vi "NI_9222_Anologue_DAQ2_FPGA_Host.vi"() -> ()   [LabVIEW 2013]
uses:
  <vilib>/rvi/interface/nirviOpenFPGA/nirviOpenFPGA.xnode
  <vilib>/rvi/interface/nirviReadWriteControl/nirviReadWriteControl.xnode
  <vilib>/rvi/interface/Simulation/niFpgaSimulationCallBeginRW.vi
  <vilib>/rvi/errors/niLvFpgaAdjustHostInterfaceError.vi
  <vilib>/rvi/interface/nirviMethod/nirviMethod.xnode
  <vilib>/rvi/errors/niLvFpgaMergeErrorWithErrorCode.vi
  <vilib>/rvi/interface/nirviCloseFPGA/nirviCloseFPGA.xnode
  <vilib>/FPGAPlugInAG/Dynamic/niLvFpga_AcknowledgeIrq_Dynamic.vi
  <vilib>/Utility/error.llb/Error Cluster From Error Code.vi
  NiFpgaLv.dll
  <vilib>/FPGAPlugInAG/Dynamic/niLvFpga_ReadFifo_Dynamic.vi
  <vilib>/rvi/interface/nirviMethod/StockFPGA_InlinedMethodWaitForSingleIRQ.vi
  <vilib>/FPGAPlugInAG/Dynamic/niLvFpga_WaitOnIrq_Dynamic.vi
  <vilib>/FPGAPlugInAG/Dynamic/niLvFpga_StartFifo_Dynamic.vi
  <vilib>/FPGAPlugInAG/Dynamic/niLvFpga_Close_Dynamic.vi
  FPGA Bitfiles/cRioProject1_FPGATarget_NI9222AnologueDA_SSoRp+cfeGo.lvbitx
  NI_9222_Anologue_DAQ2_FPGA.vi
  <vilib>/FPGAPlugInAG/cRIO-9068/niLvFpga_Open_cRIO-9068.vi
  <vilib>/rvi/interface/common/dynamic/niFpgaDynamicAddResources.vi
  <vilib>/userdefined/High Color/nirio_resource_hc.ctl
panel:
  out "Array":i16[][](array[numeric])
  out "Array Out of FIFO size":i32[](array[numeric])
  out "Array to write size":i32[](array[numeric])
  out "Number of while loop iterations":i32
  out "time string":string
  out "Elements Remaining":u32
  out "FPGA Error Out 2":errorcluster
  out "FPGA Stop":bool
  in  "RIO Device":T1="RIO0"
  out "Timed Out":bool
  out "Sample Gated":bool
  out "Overwrite":bool
  in  "stop":bool
  in  "Sample Period (uSec)":u32=2
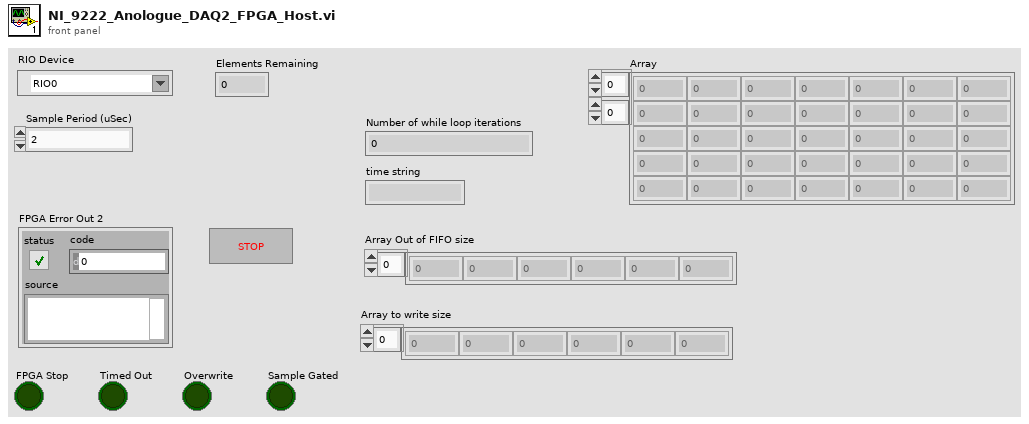
[diagram p1: front panel]
types:
  T1 = typedef "nirio_resource_hc.ctl" = tag
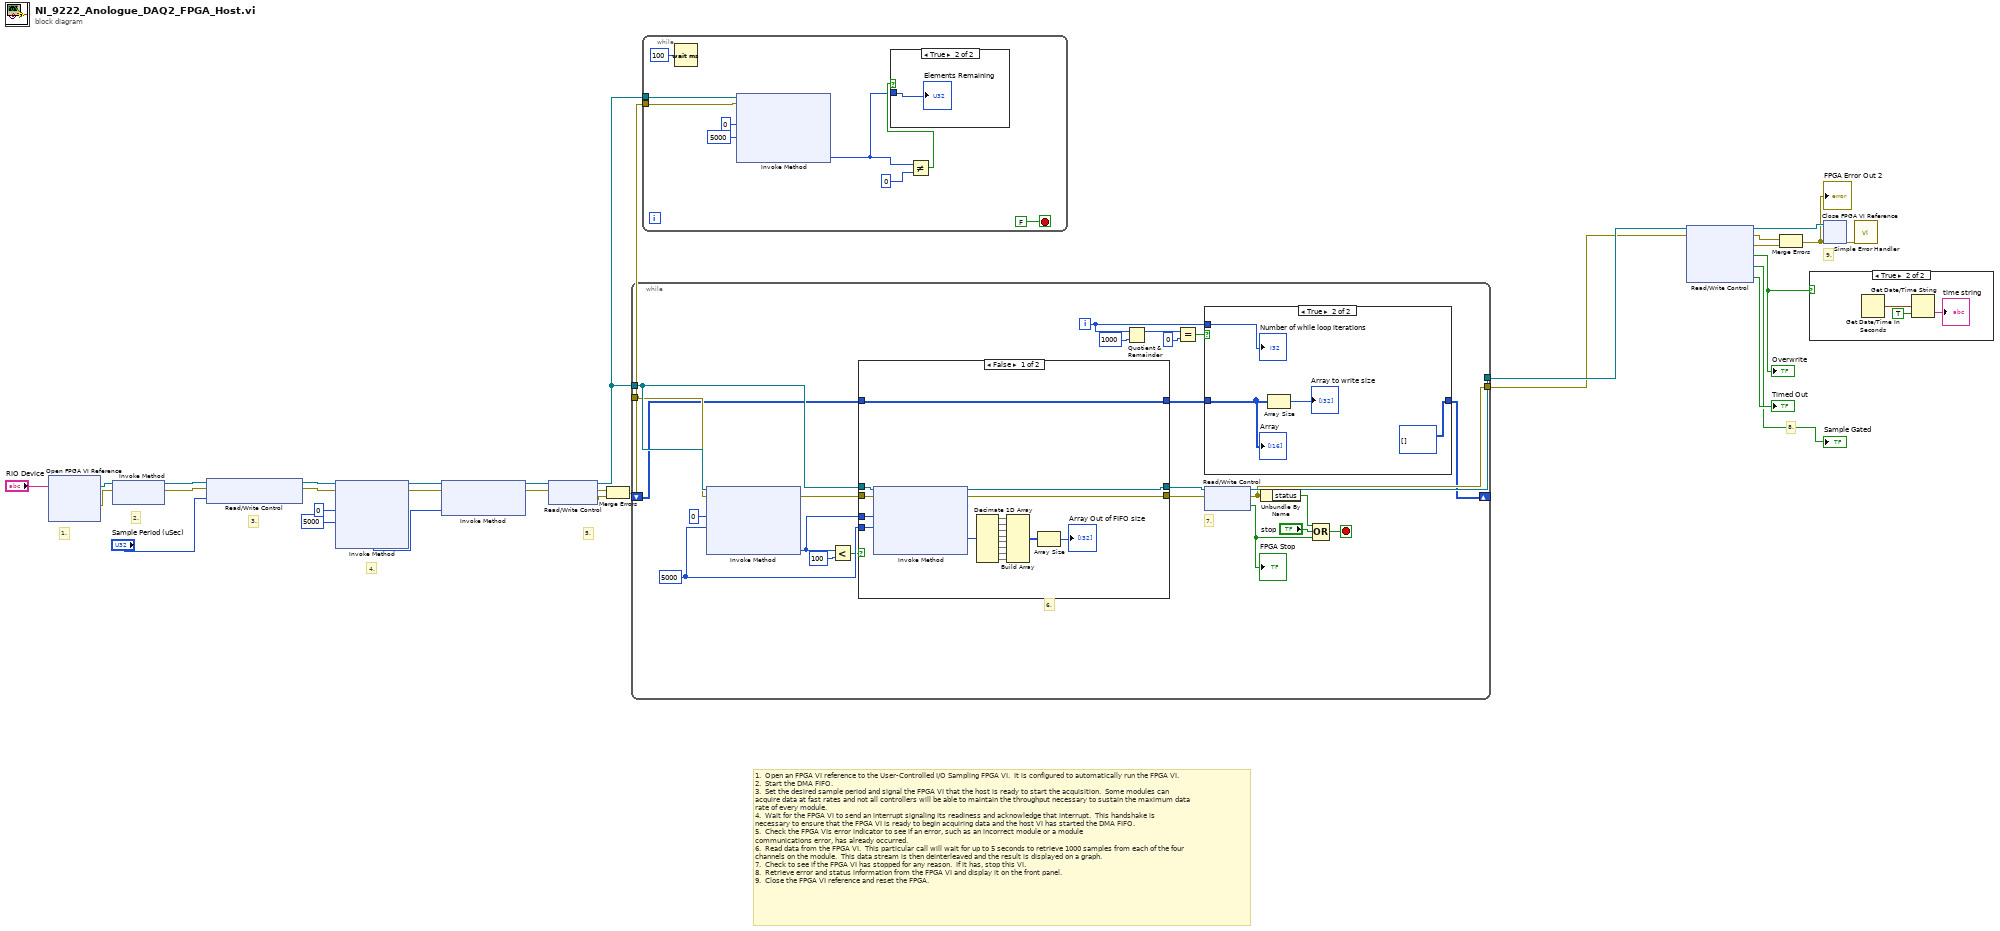
[diagram p0: block diagram]
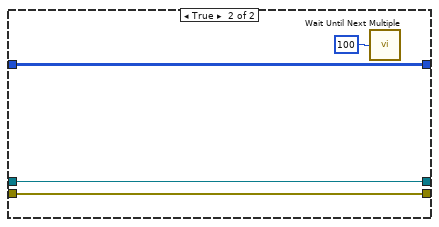
[diagram p5: hidden frame]
diagram:
  # "5."
  # "4."
  # "1.  Open an FPGA VI reference to the User-Controlled I/O Sampling FPGA VI.  It is configured to automatically run the FPGA VI.\n2.  Start the DMA FIFO.\n3.  Set the desired sample period and signal the FPGA VI that the host is ready to start the acquisition.  Some modules can \nacquire data at fast rates and not all controllers will be able to maintain the throughput necessary to sustain the maximum data \nrate of every module.\n4.  Wait for the FPGA VI to send an interrupt signaling its readiness and acknowledge that interrupt.  This handshake is \nnecessary to ensure that the FPGA VI is ready to begin acquiring data and the host VI has started the DMA FIFO.\n5.  Check the FPGA VIs error indicator to see if an error, such as an incorrect module or a module \ncommunications error, has already occurred.\n6.  Read data from the FPGA VI.  This particular call will wait for up to 5 seconds to retrieve 1000 samples from each of the four \nchannels on the module.  This data stream is then deinterleaved and the result is displayed on a graph.\n7.  Check to see if the FPGA VI has stopped for any reason.  If it has, stop this VI.\n8.  Retrieve error and status information from the FPGA VI and display it on the front panel.\n9.  Close the FPGA VI reference and reset the FPGA."
  # "9."
  # "8."
  # "3."
  # "2."
  # "1."
  n1 = xnode "Open FPGA VI Reference"("resource name"="RIO Device") -> ("FPGA VI Reference Out"=w27:refnum<k20>, "error out"=w28:errorcluster)  [unwired: 1 in]
  n2 = xnode "Invoke Method"("FPGA VI Reference In"=w27, "error in"=w28) -> ("FPGA VI Reference Out"=w26:refnum<k20>, "error out"=w25:errorcluster)
  n3 = xnode "Read/Write Control"("FPGA VI Reference In"=w26, "error in"=w25, "Sample Period (uSec)"="Sample Period (uSec)") -> ("FPGA VI Reference Out"=w13:refnum<k20>, "error out"=w12:errorcluster)
  n4 = xnode "Invoke Method"("FPGA VI Reference In"=w13, "error in"=w12, "IRQ Number(s)"=0, "Timeout (ms)"=5000) -> ("FPGA VI Reference Out"=w10:refnum<k20>, "error out"=w11:errorcluster, "IRQ(s) Asserted"=w9:i32)  [unwired: 1 out]
  n5 = xnode "Invoke Method"("FPGA VI Reference In"=w10, "error in"=w11, "IRQ Number(s)"=w9) -> ("FPGA VI Reference Out"=w5:refnum<k20>, "error out"=w4:errorcluster)
  n6 = xnode "Read/Write Control"("FPGA VI Reference In"=w5, "error in"=w4) -> ("FPGA VI Reference Out"=w3:refnum<k20>, "error out"=w15:errorcluster, "Error Out"=w14:errorcluster)
  n7 = Merge Errors(w15, w14) -> (w2:errorcluster)
  n8 = while {
    tunnel: w3 -> [w46]
    tunnel: w2 -> [w42]
    tunnel: [w52] -> w24
    tunnel: [w50] -> w23
    shift-right: [w33] -> _
    shift-left: _ -> [w30]
    i -> [w31]
    stop <- w51 stop-if-true
    w44 = 5000 ("Timeout (ms)")
    # "7."
    # "6."
    n9 = xnode "Invoke Method"("FPGA VI Reference In"=w46, "error in"=w42, "Number of Elements"=u32 0, "Timeout (ms)"=w44) -> ("error out"=w43:errorcluster, "Elements Remaining"=w38:u32)  [unwired: 2 out]
    n10 = Less?(x=w38, y=u32 100) -> (x < y?=w39:bool)
    n11 = case shown="False" w39 {
      tunnel: [w64 w80] -> w49
      tunnel: [w63 w79] -> w48
      tunnel: w46 -> [w67 w80]
      tunnel: w44 -> [w65 _]
      tunnel: w43 -> [w66 w79]
      tunnel: w38 -> [w62 _]
      tunnel: w30 -> [w61 w77]
      tunnel: [w61 w77] -> w32
      frame False {
        n12 = xnode "Invoke Method"("FPGA VI Reference In"=w67, "error in"=w66, "Number of Elements"=w62, "Timeout (ms)"=w65) -> ("FPGA VI Reference Out"=w64:refnum<k20>, "error out"=w63:errorcluster, "Data"=w68:i16[])  [unwired: 1 out]
        n13 = Decimate 1D Array(w68) -> (w72:i16[], w71:i16[], w70:i16[], w69:i16[], w73:i16[], w74:i16[], w75:i16[], w76:i16[])
        n14 = Build Array(w72, w71, w70, w69, w73, w74, w75, w76) -> (w59:i16[][])
        n15 = Array Size(array=w59) -> (size(s)=→"Array Out of FIFO size":i32[])
      }
      frame True {
        n16 = call "Wait Until Next Multiple"("Count(uSec)"=u32 100) -> ()  [unwired: 1 out]
      }
    }
    n17 = Quotient & Remainder(x=w31, y=1000) -> (x-y*floor(x/y)=w36:i32)  [unwired: 1 out]
    n18 = Equal?(x=w36, y=0) -> (x = y?=w34:bool)
    n19 = case shown="True" w34 {
      tunnel: w32 -> [w54 w57]
      tunnel: [w54 i16[][] []] -> w33
      tunnel: w31 -> [_ w55]
      frame False {
      }
      frame True {
        n20 = Array Size(array=w57) -> (size(s)=→"Array to write size":i32[])
        "Number of while loop iterations" <- w55
        "Array" <- w57
      }
    }
    n21 = xnode "Read/Write Control"("FPGA VI Reference In"=w49, "error in"=w48) -> ("FPGA VI Reference Out"=w52:refnum<k20>, "error out"=w50:errorcluster, "Stopped"=w41:bool)
    "FPGA Stop" <- w41
    n22 = Unbundle By Name(w50) -> ("status"=w53:bool)
    n23 = Compound Arithmetic op=OR(w53, "stop", w41) -> (w51:bool)
  }
  n24 = while {
    tunnel: w3 -> [w89]
    tunnel: w2 -> [w88]
    stop <- FALSE stop-if-true
    n25 = Wait (ms)(milliseconds to wait=u32 100) -> ()  [unwired: 1 out]
    n26 = xnode "Invoke Method"("FPGA VI Reference In"=w89, "error in"=w88, "Number of Elements"=u32 0, "Timeout (ms)"=5000) -> ("Elements Remaining"=w81:u32)  [unwired: 3 out]
    n27 = Not Equal?(x=w81, y=u32 0) -> (x != y?=w82:bool)
    n28 = case shown="True" w82 {
      tunnel: w81 -> [_ w90]
      frame False {
      }
      frame True {
        "Elements Remaining" <- w90
      }
    }
  }
  n29 = xnode "Read/Write Control"("FPGA VI Reference In"=w24, "error in"=w23) -> ("FPGA VI Reference Out"=w22:refnum<k20>, "error out"=w17:errorcluster, "Error Out"=w18:errorcluster, "Overwrite"=w1:bool, "Sample Gated"=→"Sample Gated":bool, "Timed Out"=→"Timed Out":bool)
  "Overwrite" <- w1
  n30 = Merge Errors(w17, w18) -> (w6:errorcluster)
  "FPGA Error Out 2" <- w6
  n31 = case shown="True" w1 {
    frame False {
    }
    frame True {
      n32 = Get Date/Time In Seconds() -> (seconds since 1Jan1904=w91:timestamp)
      n33 = Get Date/Time String(seconds (now)=w91, want seconds? (F)=TRUE) -> (time string=→"time string":string)  [unwired: 1 in, 1 out]
    }
  }
  n34 = xnode "Close FPGA VI Reference"("FPGA VI Reference In"=w22, "error in"=w6) -> ("error out"=w16:errorcluster)
  n35 = call <vilib>:"Simple Error Handler.vi"("error in (no error)"=w16) -> ()  [unwired: 4 in, 5 out]
